vi "GetBinnedData.vi"(0 "VISA resource name":refnum<visa-resource-name>, 1 "Show on call?":bool=TRUE, 3 "Maximum Value":dbl=1.5e-07 format="%#_13g", 5 "Time in ms (30000)":u32=30000, 9 "Time between calibrations (ms)":u32=1000, 11 "error in":errorcluster, 12 "# bins":i32, 14 "Minimum Value":dbl format="%#_13g") -> (4 "VISA resource name out":refnum<visa-resource-name>, 6 "Binned time":dbl[](array[numeric]), 10 "Unbinned times / s":dbl[](array[numeric]), 15 "error out":errorcluster)   [LabVIEW 2017, in "GP22_TDC_Arduinoed.lvlib"]
doc: "Get data in the format that the ORTEC used to output. \n\nThis VI will take measurements for a given amount of time, bin the timings and output an array of the binned data."
uses:
  GP22_TDC_Arduinoed.lvlib
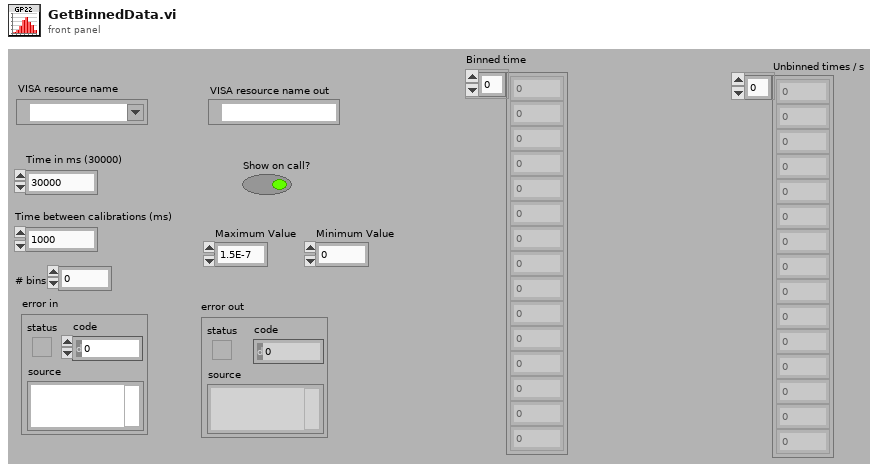
[diagram p1: front panel]
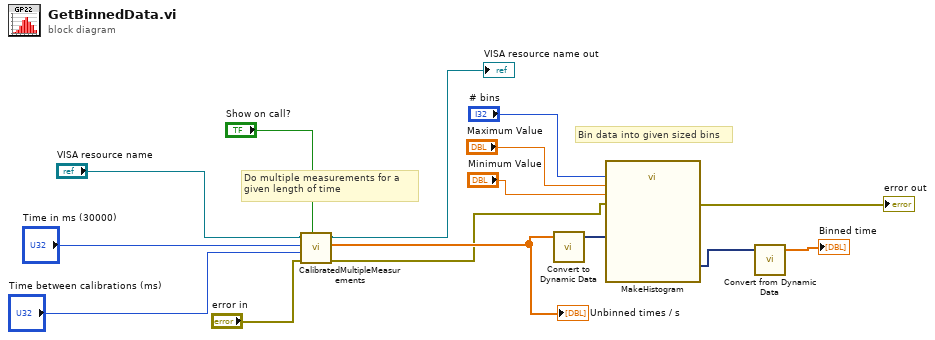
[diagram p0: block diagram]
diagram:
  # "Bin data into given sized bins"
  # "Do multiple measurements for a \ngiven length of time"
  n1 = call "CalibratedMultipleMeasurements.vi"("Show on call?"="Show on call?", "error in"="error in", "Time between calibrations (ms)"="Time between calibrations (ms)", "Time / ms (30000)"="Time in ms (30000)", "VISA resource name"="VISA resource name") -> ("error out"=w5:errorcluster, "Times / s"=w9:dbl[], "VISA resource name out"=→"VISA resource name out":refnum<visa-resource-name>)  [unwired: 3 in, 1 out]
  "Unbinned times / s" <- w9
  n2 = call "Convert to Dynamic Data"("Array"=w9) -> ("Dynamic Data Type"=w8:dynamicdata)  [unwired: 3 in]
  n3 = call "MakeHistogram.vi"("Signal"=w8, "Number of Bins"="# bins", "Maximum Value"="Maximum Value", "Minimum Value"="Minimum Value", "error in (no error)"=w5) -> ("Histogram"=w2:dynamicdata, "error out"=→"error out":errorcluster)  [unwired: 9 in]
  n4 = call "Convert from Dynamic Data"("Dynamic Data Type"=w2) -> ("Array"=→"Binned time":dbl[])  [unwired: 3 in]
